vi "HexapodCloseHardware.vi"(8 "error in (no error)":errorcluster, 11 "HexapodPI in":refnum<class "HexapodPI.lvclass">) -> (0 "error out":errorcluster)   [LabVIEW 2020, in "HexapodPI.lvclass"]
uses:
  HexapodPI.lvclass
  HexapodPI.lvclass/HexapodPI.ctl
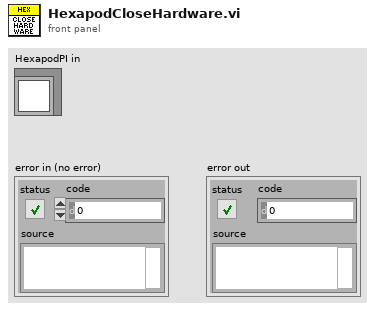
[diagram p1: front panel]
types:
  T1 = typedef "OnOffTypeDef.ctl" = enum16{"off", "on"}
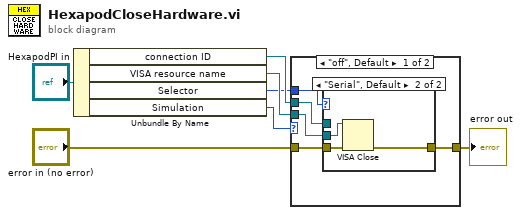
[diagram p0: block diagram]
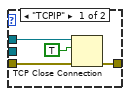
[diagram p2: hidden frame]
diagram:
  n1 = Unbundle By Name("HexapodPI in") -> ("connection ID"=w5:refnum<k5>, "VISA resource name"=w6:refnum<visa-resource-name>, "Selector"=w4:enum16{"TCPIP", "Serial"}, "Simulation"=w7:T1)
  n2 = case shown="\"off\", Default" w7 {
    tunnel: "error in (no error)" -> [w12 w20]
    tunnel: [w11 w20] -> w3
    tunnel: w4 -> [w10 _]
    tunnel: w5 -> [w9 _]
    tunnel: w6 -> [w8 _]
    frame "off", Default {
      n3 = case shown="\"Serial\", Default" w10 {
        tunnel: w12 -> [w15 w18]
        tunnel: [w14 w17] -> w11
        tunnel: w9 -> [w13 _]
        tunnel: w8 -> [_ w19]
        frame "TCPIP" {
          n4 = TCP Close Connection(connection ID=w13, abort (F)=TRUE, error in (no error)=w15) -> (error out=w14:errorcluster)  [unwired: 1 out]
        }
        frame "Serial", Default {
          n5 = VISA Close(VISA resource name=w19, error in (no error)=w18) -> (error out=w17:errorcluster)
        }
      }
    }
    frame "on" {
    }
  }
  "error out" <- w3
